vi "ControlYaw.vi"() -> ()   [LabVIEW 2014]
uses:
  <vilib>/LVH/AR Drone Toolkit/Decode NavData/Typedefs/NavData Demo.ctl
  <vilib>/Utility/inputDevices.llb/closeJoystick.vi
  <vilib>/LVH/AR Drone Toolkit/AR Drone.lvlib
panel:
  out "Altura Cm":dbl
  in  "SetAltura":u32(knob) scale=15.0..100.0
  in  "Angulo":i16(knob) scale=0.0..360.0
  out "Gamepad Output":T1
  out "NavData Out":T2
  out "Battery Remaining":dbl(slide) scale=0.0..100.0
  in  "stop":bool
  out "Axes Output":T3 {"Vertical Speed" scale=-1.0..1.0; "Yaw Speed" scale=-1.0..1.0; "Pitch" scale=-1.0..1.0; "Roll" scale=-1.0..1.0}
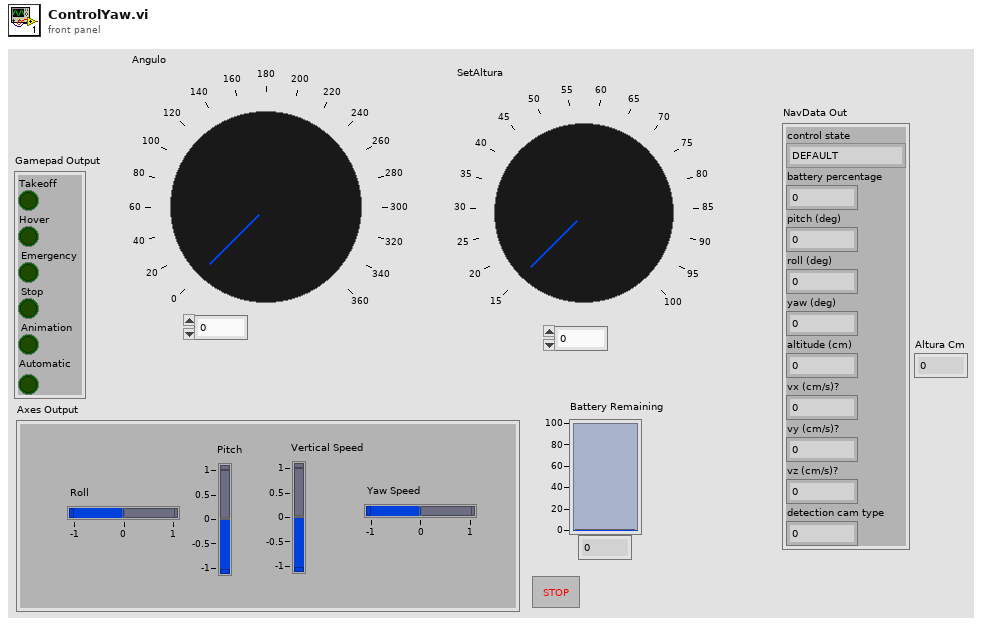
[diagram p1: front panel]
types:
  T1 = cluster{"Takeoff":bool, "Hover":bool, "Emergency":bool, "Stop":bool, "Animation":bool, "Automatic":bool}
  T2 = typedef "AR Drone.lvlib/NavData Demo.ctl" = cluster{"control state":enum32{"DEFAULT", "INIT", "LANDING", "FLYING", "HOVERING", "TEST", "TRANS_TAKEOFF", "TRANS_GOTOFIX", "TRANS_LANDING"}, "battery percentage":u32, "pitch (deg)":sgl, "roll (deg)":sgl, "yaw (deg)":sgl, "altitude (cm)":u32, "vx (cm/s)?":sgl, "vy (cm/s)?":sgl, "vz (cm/s)?":sgl, "detection cam type":u32}
  T3 = cluster{"Roll":dbl, "Pitch":dbl, "Vertical Speed":dbl, "Yaw Speed":dbl}
  T4 = typedef "AR Drone.lvlib/AR Drone Resource.ctl" = cluster{"UDP Control Connection":refnum<k16>, "UDP NavData Connection":refnum<k16>, "UDP Video Connection (Drone 1.0)":refnum<k16>, "TCP Video Connection (Drone 2.0)":refnum<k5>, "TCP Control Port Connection":refnum<k5>, "Drone IP address":string, "Drone Command Port":u16, "Drone NavData Port":u16, "Drone Vid Stream Port":u16, "Drone TCP Control Port":u16, "Home IP address":string, "Home Command Port":u16, "Home NavData Port":u16, "Home Vid Stream Port":u16, "Drone Version":i32}
  T5 = cluster{"Roll":sgl, "Pitch":sgl, "Vertical Speed":sgl, "Yaw Speed":sgl}
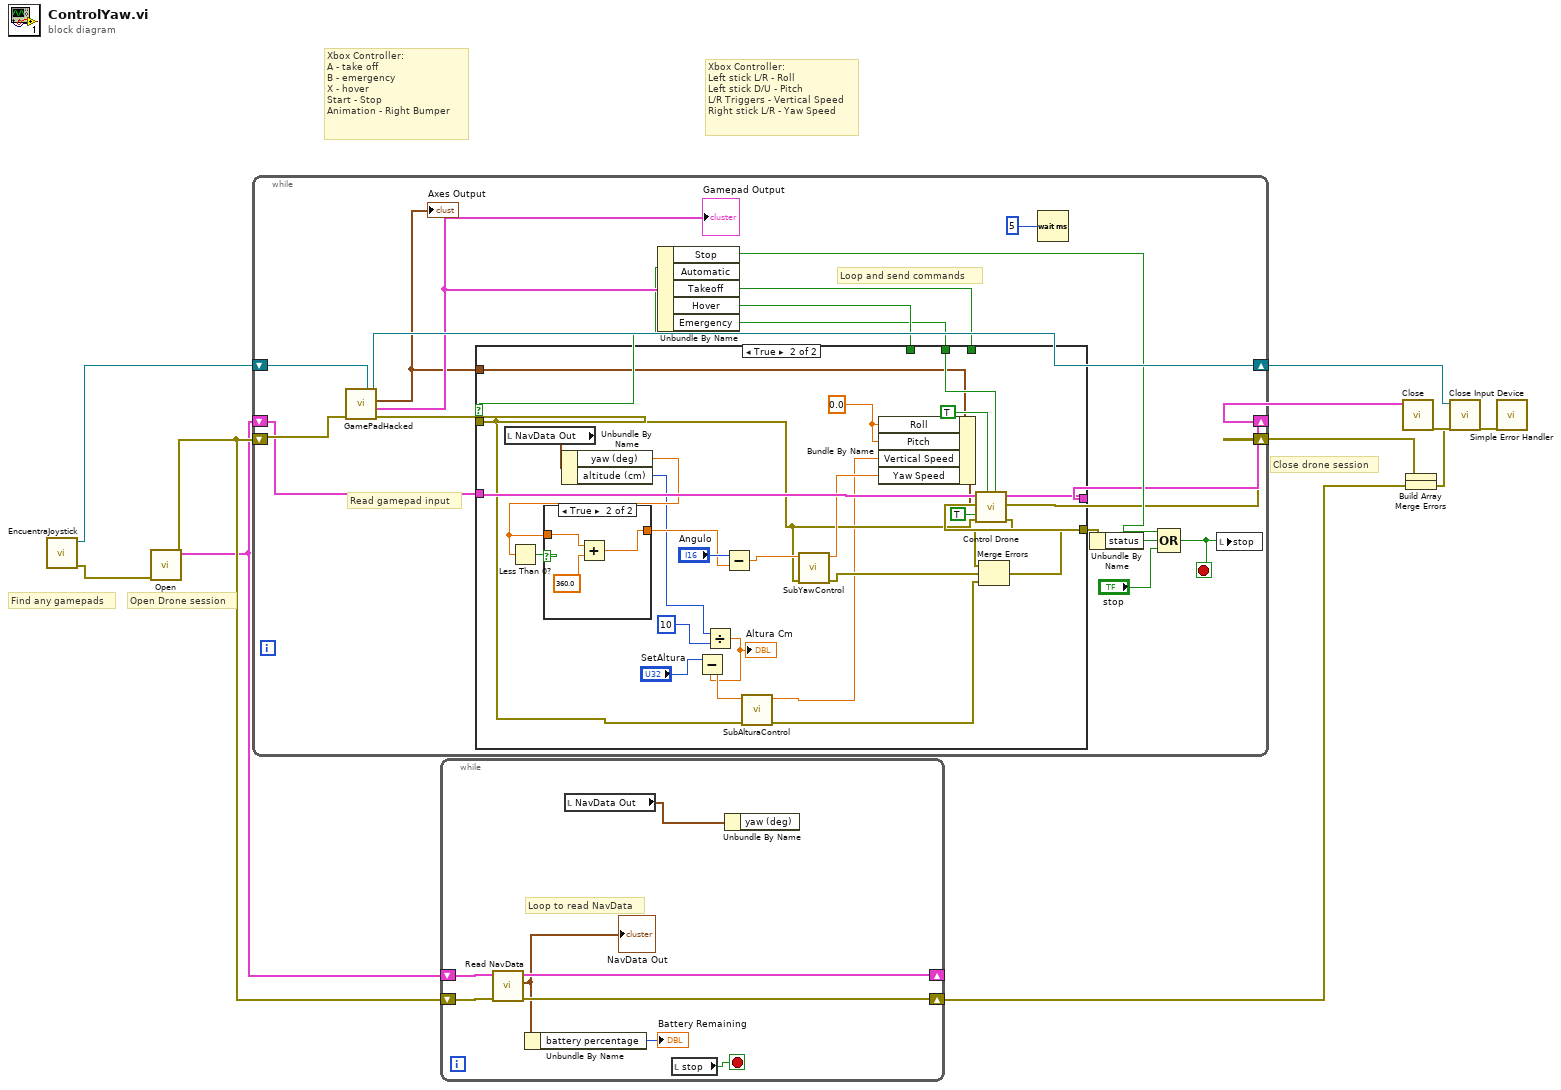
[diagram p0: block diagram]
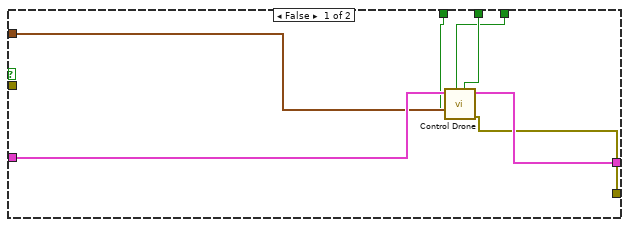
[diagram p2: hidden frame]
diagram:
  # "Close drone session"
  # "Open Drone session"
  # "Find any gamepads"
  # "Xbox Controller:\nLeft stick L/R - Roll\nLeft stick D/U - Pitch\nL/R Triggers - Vertical Speed\nRight stick L/R - Yaw Speed"
  # "Xbox Controller:\nA - take off\nB - emergency\nX - hover\nStart - Stop\nAnimation - Right Bumper"
  n1 = call "EncuentraJoystick.vi"() -> ("error out"=w1:errorcluster, "Refnum out"=w2:refnum<k1>)  [unwired: 10 in]
  n2 = call <vilib>:"Open.vi"("error in (no error)"=w1) -> ("error out"=w5:errorcluster, "AR Drone Resource"=w3:T4)  [unwired: 9 in]
  n3 = while {
    shift-right: [w19] -> w12
    shift-left: w3 -> [w20]
    shift-right: [w18] -> w7
    shift-left: w5 -> [w24]
    shift-right: [w27] -> w11
    shift-left: w2 -> [w26]
    stop <- w28 stop-if-true
    # "Loop and send commands"
    # "Read gamepad input"
    n4 = call "GamePadHacked.vi"("error in (no error)"=w24, "Refnum in"=w26) -> ("error out"=w13:errorcluster, "Gamepad Output"=w23:T1, "Control Cluster"=w14:T5, "Refnum out"=w27:refnum<k1>)  [unwired: 6 in]
    "Axes Output" <- w14
    "Gamepad Output" <- w23
    n5 = Unbundle By Name(w23) -> ("Stop"=w21:bool, "Automatic"=w22:bool, "Takeoff"=w17:bool, "Hover"=w16:bool, "Emergency"=w15:bool)
    n6 = case shown="True" w22 {
      tunnel: [w35 w52] -> w18
      tunnel: w20 -> [w36 w63]
      tunnel: [w37 w61] -> w19
      tunnel: w17 -> [w32 _]
      tunnel: w16 -> [w31 _]
      tunnel: w15 -> [w33 w62]
      tunnel: w14 -> [w34 w56]
      tunnel: w13 -> [_ w41]
      frame False {
        n7 = call <vilib>:"Control Drone.vi"("Emergency Landing"=w33, "Takeoff/Land"=w32, "Hover"=w31, "Control Cluster"=w34, "AR Drone Resource"=w36) -> ("error out"=w35:errorcluster, "AR Drone Resource Out"=w37:T4)  [unwired: 5 in]
      }
      frame True {
        w55 = sgl 0.0 ("Roll")
        n8 = local read "NavData Out"() -> (w58:T2)
        n9 = Unbundle By Name(w58) -> ("yaw (deg)"=w47:sgl, "altitude (cm)"=w38:u32)
        n10 = Less Than 0?(x=w47) -> (x < 0?=w48:bool)
        n11 = case shown="True" w48 {
          tunnel: w47 -> [w64 w67]
          tunnel: [w64 w65] -> w46
          frame False {
          }
          frame True {
            n12 = Add(x=w67, y=sgl 360.0) -> (x+y=w65:sgl)
          }
        }
        n13 = Divide(x=w38, y=u32 10) -> (x/y=w43:dbl)
        "Altura Cm" <- w43
        n14 = Subtract(x="SetAltura", y=w43) -> (x-y=w44:dbl)
        n15 = Subtract(x="Angulo", y=w46) -> (x-y=w50:sgl)
        n16 = call "SubAlturaControl.vi"("error in (no error)"=w41, "input value"=w44) -> ("error out"=w40:errorcluster, "output value"=w39:dbl)  [unwired: 8 in]
        n17 = call "SubYawControl.vi"("error in (no error)"=w41, "input value"=w50) -> ("error out"=w53:errorcluster, "output value"=w51:dbl)  [unwired: 8 in]
        n18 = Bundle By Name(cluster=w56, "Roll"=w55, "Pitch"=w55, "Vertical Speed"=w39, "Yaw Speed"=w51) -> (w57:T5)
        n19 = call <vilib>:"Control Drone.vi"("Emergency Landing"=w62, "Takeoff/Land"=TRUE, "error in (no error)"=w41, "Hover"=TRUE, "Control Cluster"=w57, "AR Drone Resource"=w63) -> ("error out"=w54:errorcluster, "AR Drone Resource Out"=w61:T4)  [unwired: 4 in]
        n20 = Merge Errors(w54, w53, w40) -> (w52:errorcluster)
      }
    }
    n21 = Wait (ms)(milliseconds to wait=u32 5) -> ()  [unwired: 1 out]
    n22 = Unbundle By Name(w18) -> ("status"=w25:bool)
    n23 = Compound Arithmetic op=OR(w21, w25, "stop") -> (w28:bool)
    n24 = local write "stop"(w28) -> ()
  }
  n25 = while {
    shift-right: [w74] -> _
    shift-left: w3 -> [w75]
    shift-right: [w72] -> w6
    shift-left: w5 -> [w73]
    stop <- w69 stop-if-true
    # "Loop to read NavData"
    n26 = call <vilib>:"Read NavData.vi"("error in (no error)"=w73, "AR Drone Resource"=w75) -> ("error out"=w72:errorcluster, "NavData Out"=w71:T2, "AR Drone Resource Out"=w74:T4)  [unwired: 7 in]
    "NavData Out" <- w71
    n27 = Unbundle By Name(w71) -> ("battery percentage"=→"Battery Remaining":u32)
    n28 = local read "NavData Out"() -> (w68:T2)
    n29 = local read "stop"() -> (w69:bool)
    n30 = Unbundle By Name(w68) -> ()  [unwired: 1 out]
  }
  n31 = Build Array(w7, w6) -> (w4:errorcluster[])
  n32 = Merge Errors(w4) -> (w8:errorcluster)
  n33 = call <vilib>:"Close.vi"("error in (no error)"=w8, "AR Drone Resource"=w12) -> ("error out"=w10:errorcluster)  [unwired: 9 in]
  n34 = call-poly <vilib>:"Close Input Device.vi"("error in (no error)"=w10, "device ID"=w11) -> ("error out"=w9:errorcluster)  [unwired: 8 in]
  n35 = call <vilib>:"Simple Error Handler.vi"("error in (no error)"=w9) -> ()  [unwired: 4 in, 5 out]
